vi "DSF.Engine.Plugin.Parse Command.Transfer Group.vi"(8 "error in (no error)":errorcluster, 10 "Command Parameters":T1, 11 "Plugin in":refnum<class "Plugin.lvclass">) -> (0 "error out":errorcluster, 2 "transfer group id":i32, 3 "Plugin out":refnum<class "Plugin.lvclass">)   [LabVIEW 2017, in "DSF.Engine.lvlib" / "Plugin.lvclass"]
uses:
  Plugin.lvclass
  Interface/DSF.Engine.Interface.Plugin.Command Parameters.ctl
  Interface/DSF.Engine.Interface.Plugin.lvclass
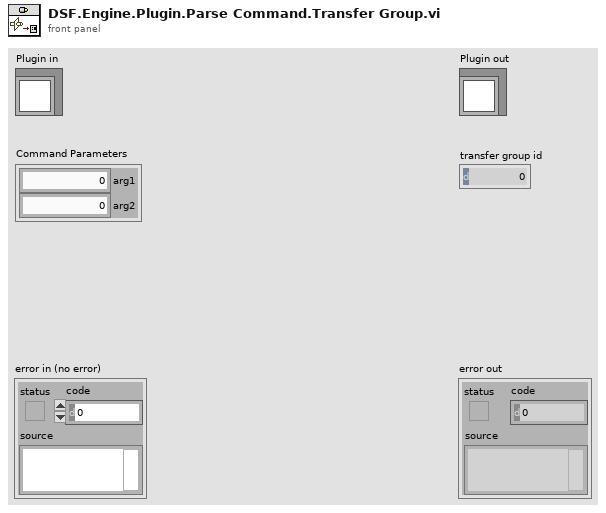
[diagram p1: front panel]
types:
  T1 = typedef "DSF.Engine.lvlib/DSF.Engine.Interface.Plugin.lvclass/DSF.Engine.Interface.Plugin.Command Parameters.ctl" = cluster{"arg1":u64, "arg2":u64}
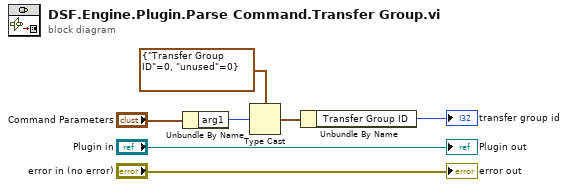
[diagram p0: block diagram]
diagram:
  n1 = Unbundle By Name("Command Parameters") -> ("arg1"=w5:u64)
  n2 = Type Cast(type=cluster{"Transfer Group ID":i32, "unused":i32} {"Transfer Group ID"=0, "unused"=0}, x=w5) -> (*(type *) &x=w4:cluster{"Transfer Group ID":i32, "unused":i32})
  n3 = Unbundle By Name(w4) -> ("Transfer Group ID"=→"transfer group id":i32)
  "error out" <- "error in (no error)"
  "Plugin out" <- "Plugin in"
